vi "UDP Packet Preferences.vi"(9 "Named Controls in":T1, 10 "Operation":enum16{"Save", "Load"}(ring)=enum."Load", 11 "Refnum":T2) -> (2 "Count":i32, 3 "Warnings List":string)   [LabVIEW 2013]
uses:
  <vilib>/Utility/config.llb/Config Data RefNum.ctl
  Named Control.ctl
  <vilib>/Utility/config.llb/NI_LVConfig.lvlib
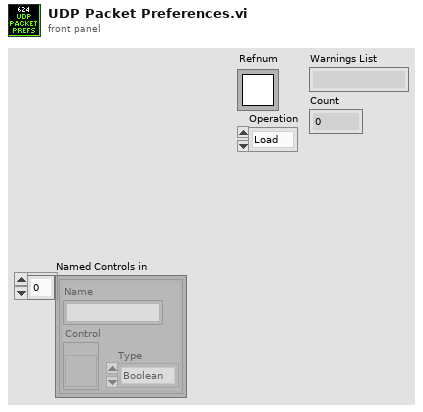
[diagram p1: front panel]
types:
  T1 = typedef "Named Control.ctl" = cluster{"Name":string, "Control":refnum<vi>, "Type":enum16{"Boolean", "Double"}}[]
  T2 = typedef "NI_LVConfig.lvlib/Config Data RefNum.ctl" = refnum<k1>
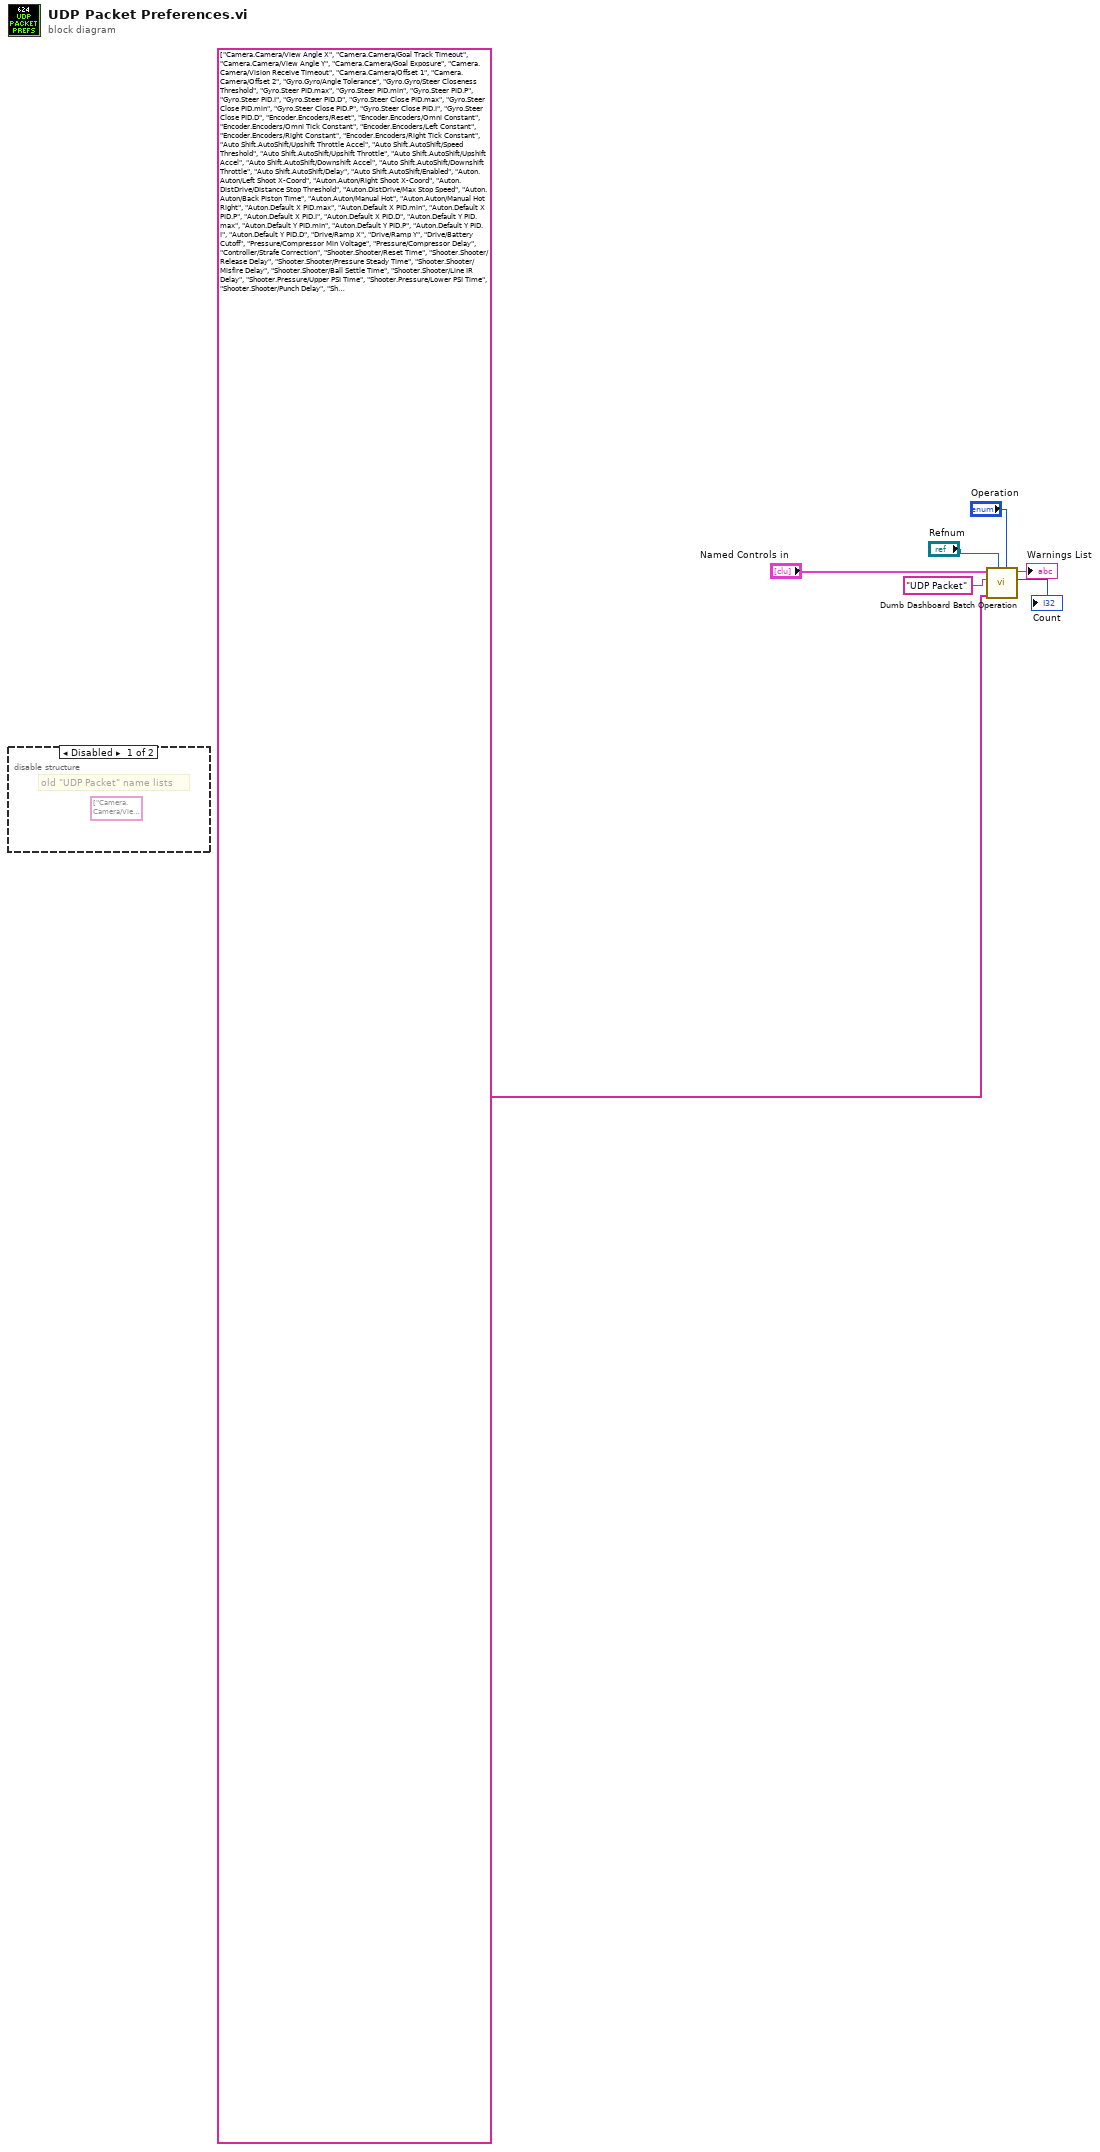
[diagram p0: block diagram]
diagram:
  n1 = disable-structure shown="Disabled" {
    frame Disabled {
      (unwired) string[] ["Camera.Camera/View Angle X", "Camera.Camera/Goal Track Timeout", "Camera.Camera/View Angle Y", "Camera.Camera/Goal Exposure", "Camera.Camera/Vision Receive Timeout", "Camera.Camera/Offset 1", "Camera.Camera/Offset 2", "Gyro.Gyro/Angle Tolerance", "Gyro.Gyro/Steer Closeness Threshold", "Gyro.Steer PID.max", "Gyro.Steer PID.min", "Gyro.Steer PID.P", "Gyro.Steer PID.I", "Gyro.Steer PID.D", "Gyro.Steer Close PID.max", "Gyro.Steer Close PID.min", "Gyro.Steer Close PID.P", "Gyro.Steer Close PID.I", "Gyro.Steer Close PID.D", "Encoder.Encoders/Reset", "Encoder.Encoders/Omni Constant", "Encoder.Encoders/Omni Tick Constant", "Encoder.Encoders/Left Constant", "Encoder.Encoders/Right Constant", "Encoder.Encoders/Right Tick Constant", "Auto Shift.AutoShift/Upshift Throttle Accel", "Auto Shift.AutoShift/Speed Threshold", "Auto Shift.AutoShift/Upshift Throttle", "Auto Shift.AutoShift/Upshift Accel", "Auto Shift.AutoShift/Downshift Accel", "Auto Shift.AutoShift/Downshift Throttle", "Auto Shift.AutoShift/Delay", "Auto Shift.AutoShift/Enabled", "Auton.Auton/Left Shoot X-Coord", "Auton.Auton/Right Shoot X-Coord", "Auton.DistDrive/Distance Stop Threshold", "Auton.DistDrive/Max Stop Speed", "Auton.Auton/Back Piston Time", "Auton.Auton/Manual Hot", "Auton.Auton/Manual Hot Right", "Auton.Default X PID.max", "Auton.Default X PID.min", "Auton.Default X PID.P", "Auton.Default X PID.I", "Auton.Default X PID.D", "Auton.Default Y PID.max", "Auton.Default Y PID.min", "Auton.Default Y PID.P", "Auton.Default Y PID.I", "Auton.Default Y PID.D", "Drive/Ramp X", "Drive/Ramp Y", "Drive/Battery Cutoff", "Pressure/Compressor Min Voltage", "Pressure/Compressor Delay", "Controller/Strafe Correction", "Shooter.Shooter/Reset Time", "Shooter.Shooter/Release Delay", "Shooter.Shooter/Pressure Steady Time", "Shooter.Shooter/Misfire Delay", "Shooter.Shooter/Ball Settle Time", "Shooter.Shooter/Line IR Delay", "Shooter.Pressure/Upper PSI Time", "Shooter.Pressure/Lower PSI Time", "Shooter.Shooter/Punch Delay", "Shooter.Shooter/Target Pressure", "Shooter.Pressure/Line B", "Shooter.Pressure/Line M", "Shooter.Pressure/Shooter M", "Shooter.Pressure/Shooter B", "Rollers.Roller/Load IRs Verify Time", "Rollers.Roller/Center IR Latch Time", "Rollers.Roller/Speed Front", "Rollers.Roller/Speed Back", "Rollers.Roller/Entry Timeout", "Rollers.Roller/To Center Timeout", "Rollers.Roller/Sustain Time", "Rollers.Roller/Verify Center Time", "Abort", "Finish", "Shooter Halo Time", "IR Halo Sustain Time", "Disable Compressor"]
      # "old \"UDP Packet\" name lists"
    }
    frame Enabled {
    }
  }
  n2 = call "Dumb Dashboard Batch Operation.vi"("Operation"="Operation", "Refnum in"="Refnum", "Names List"=string[] ["Camera.Camera/View Angle X", "Camera.Camera/Goal Track Timeout", "Camera.Camera/View Angle Y", "Camera.Camera/Goal Exposure", "Camera.Camera/Vision Receive Timeout", "Camera.Camera/Offset 1", "Camera.Camera/Offset 2", "Gyro.Gyro/Angle Tolerance", "Gyro.Gyro/Steer Closeness Threshold", "Gyro.Steer PID.max", "Gyro.Steer PID.min", "Gyro.Steer PID.P", "Gyro.Steer PID.I", "Gyro.Steer PID.D", "Gyro.Steer Close PID.max", "Gyro.Steer Close PID.min", "Gyro.Steer Close PID.P", "Gyro.Steer Close PID.I", "Gyro.Steer Close PID.D", "Encoder.Encoders/Reset", "Encoder.Encoders/Omni Constant", "Encoder.Encoders/Omni Tick Constant", "Encoder.Encoders/Left Constant", "Encoder.Encoders/Right Constant", "Encoder.Encoders/Right Tick Constant", "Auto Shift.AutoShift/Upshift Throttle Accel", "Auto Shift.AutoShift/Speed Threshold", "Auto Shift.AutoShift/Upshift Throttle", "Auto Shift.AutoShift/Upshift Accel", "Auto Shift.AutoShift/Downshift Accel", "Auto Shift.AutoShift/Downshift Throttle", "Auto Shift.AutoShift/Delay", "Auto Shift.AutoShift/Enabled", "Auton.Auton/Left Shoot X-Coord", "Auton.Auton/Right Shoot X-Coord", "Auton.DistDrive/Distance Stop Threshold", "Auton.DistDrive/Max Stop Speed", "Auton.Auton/Back Piston Time", "Auton.Auton/Manual Hot", "Auton.Auton/Manual Hot Right", "Auton.Default X PID.max", "Auton.Default X PID.min", "Auton.Default X PID.P", "Auton.Default X PID.I", "Auton.Default X PID.D", "Auton.Default Y PID.max", "Auton.Default Y PID.min", "Auton.Default Y PID.P", "Auton.Default Y PID.I", "Auton.Default Y PID.D", "Drive/Ramp X", "Drive/Ramp Y", "Drive/Battery Cutoff", "Pressure/Compressor Min Voltage", "Pressure/Compressor Delay", "Controller/Strafe Correction", "Shooter.Shooter/Reset Time", "Shooter.Shooter/Release Delay", "Shooter.Shooter/Pressure Steady Time", "Shooter.Shooter/Misfire Delay", "Shooter.Shooter/Ball Settle Time", "Shooter.Shooter/Line IR Delay", "Shooter.Pressure/Upper PSI Time", "Shooter.Pressure/Lower PSI Time", "Shooter.Shooter/Punch Delay", "Shooter.Shooter/Target Pressure", "Shooter.Pressure/Line B", "Shooter.Pressure/Line M", "Shooter.Pressure/Shooter M", "Shooter.Pressure/Shooter B", "Shooter.Halo Time", "Shooter.Soft Release Delay", "Shooter.Soft Unpin Delay", "Shooter.Soft Shoot Delay", "Rollers.Roller/Load IRs Verify Time", "Rollers.Roller/Center IR Latch Time", "Rollers.Roller/Speed Front", "Rollers.Roller/Speed Back", "Rollers.Roller/Entry Timeout", "Rollers.Roller/To Center Timeout", "Rollers.Roller/Sustain Time", "Rollers.Roller/Verify Center Time", "Abort", "Finish", "IR Halo Sustain Time", "Disable Compressor", "Center Omni Drive Delay", "Radius Throttle", "Fieldcentric.X/Y ratio low", "Fieldcentric.X/Y ratio high", "Fieldcentric.Steering Gain", "Fieldcentric.Enable", "Fieldcentric.Relative Angle", "Fieldcentric.Point Robot", "Fieldcentric.Force Omni Down", "Roll.X 1", "Roll.Y 1", "Roll.X 2", "Roll.Y 2", "Roll.X 3", "Roll.Y 3", "Roll.Time 1", "Roll.Time 2", "Roll.Time 3", "Roll.Angle Start", "Roll.Angle End", "Roll.Angle Linearity", "Stick Deadband", "Auton.Half Over Delay", "Shooter.Toss Release Time"], "Section"="UDP Packet", "Named Controls in"="Named Controls in") -> ("Count"=→"Count":i32, "Warnings List"=→"Warnings List":string)  [unwired: 5 in]
